vi "translatePolarityValues.vi"(0 "SingleAxisController in":refnum<class "_SingleAxisController.lvclass">, 1 "simple_actions":T3, 2 "polarity_value (in)":u32, 3 "polarity_items (in)":T1[](array[typedef]), 5 "error in (no error)":errorcluster) -> (14 "SingleAxisController out":refnum<class "_SingleAxisController.lvclass">, 16 "polarity_value (out)":u32, 17 "polarity_items (out)":T1[](array[typedef]), 19 "error out":errorcluster)   [LabVIEW 2020, in "classes.lvlib" / "_SingleAxisController.lvclass"]
doc: "Produced By:\n\n<B>Kod Integrations, LLC</B>\n4835 Marianne Drive\nMount Airy, MD 21771\nhttp://www.kodintegrations.com\nemail: info@kodintegrations.com\nphone: (240) 687-1288"
uses:
  _SingleAxisController.lvclass
  common/controls/simple_actions.ctl
  common/controls/polarity_item.ctl
  common/controls/polarity.ctl
  libraries/common.lvlib
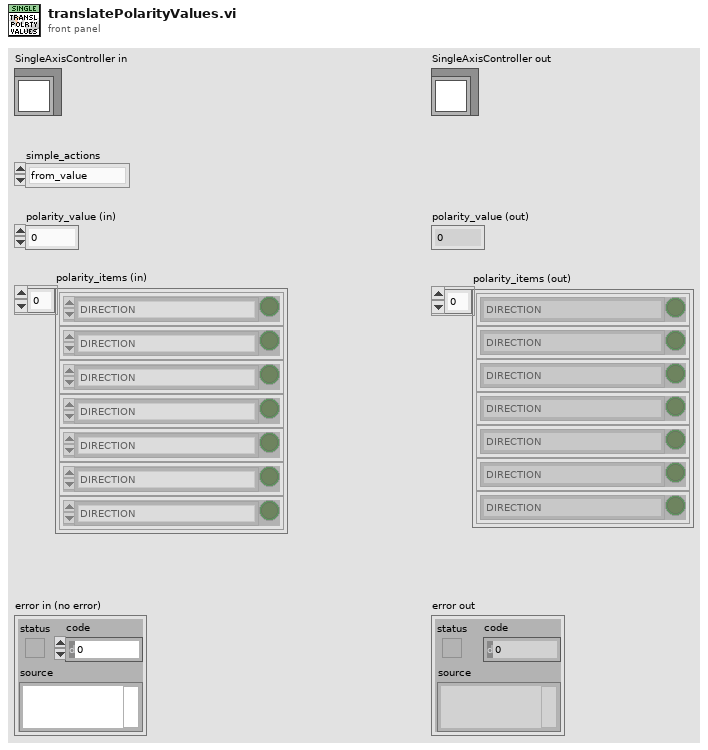
[diagram p1: front panel]
types:
  T1 = typedef "common.lvlib/polarity_item.ctl" = cluster{"item":T2, "status":bool}
  T2 = typedef "common.lvlib/polarity.ctl" = enum16{"DIRECTION", "LIMIT", "HOME", "DIG_OUT", "DIG_IN", "ENABLE_OUT", "JUMP_ERR", "LATCH", "Z-CHAN_INDEX", "ENCODER_DECODING:1X", "ENCODER_DECODING:2X", "ENCODER_DECODING:4X", "ALARM", "STANDALONE_ERR", "-", "<reserved/nc>"}
  T3 = typedef "common.lvlib/simple_actions.ctl" = enum16{"from_value", "to_value"}
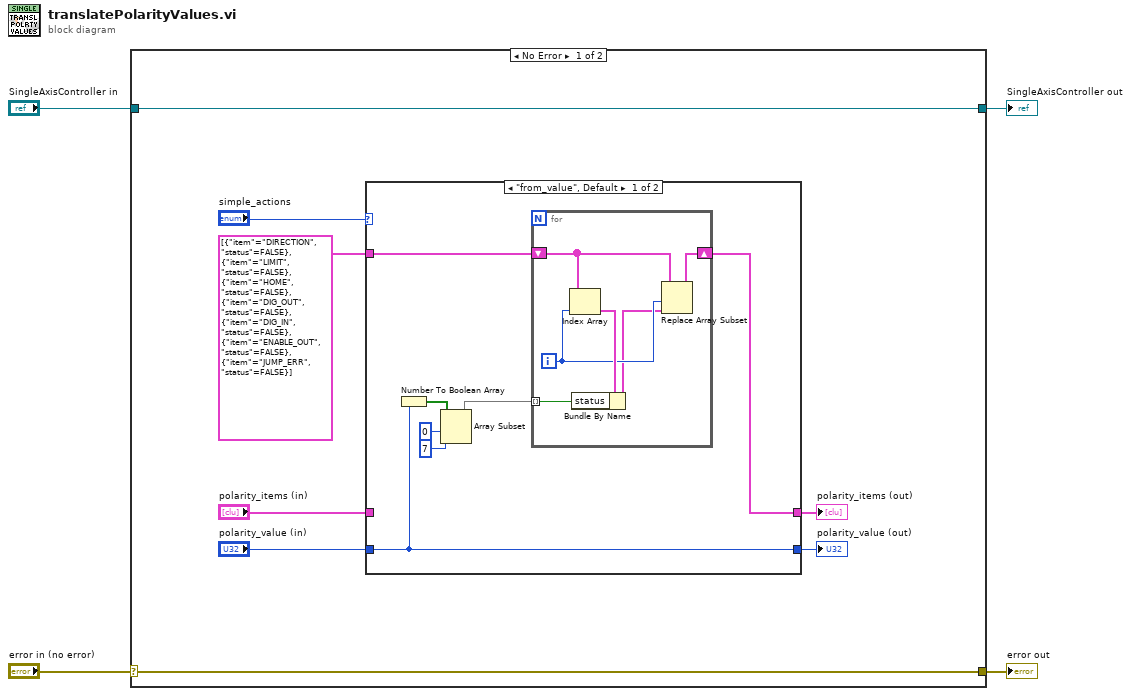
[diagram p0: block diagram]
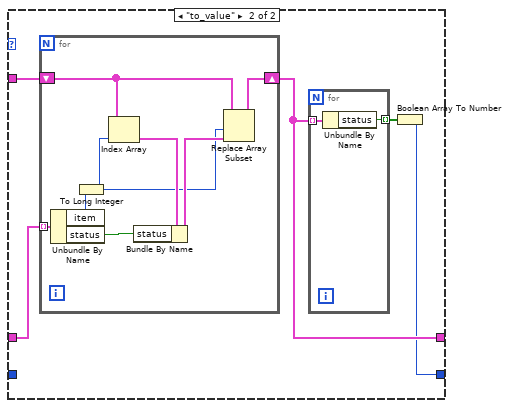
[diagram p2: hidden frame]
diagram:
  n1 = case shown="No Error" "error in (no error)" {
    selector: "error in (no error)" -> [w11 w42]
    tunnel: [w11 w42] -> w3
    tunnel: [w12 w41] -> w1
    tunnel: "SingleAxisController in" -> [w12 w41]
    frame No Error {
      n2 = case shown="\"from_value\", Default" "simple_actions" {
        tunnel: "polarity_value (in)" -> [w13 _]
        tunnel: [w15 w28] -> w8
        tunnel: T1[] [{"item"=enum."DIRECTION", "status"=FALSE}, {"item"=enum."LIMIT", "status"=FALSE}, {"item"=enum."HOME", "status"=FALSE}, {"item"=enum."DIG_OUT", "status"=FALSE}, {"item"=enum."DIG_IN", "status"=FALSE}, {"item"=enum."ENABLE_OUT", "status"=FALSE}, {"item"=enum."JUMP_ERR", "status"=FALSE}] ("polarity_items (in)") -> [w14 w30]
        tunnel: "polarity_items (in)" -> [_ w29]
        tunnel: [w13 w26] -> w5
        frame "from_value", Default {
          n3 = Number To Boolean Array(number=w13) -> (Boolean array=w19:bool[])
          n4 = Array Subset(array=w19, index=0, length=7) -> (w16:bool[])
          n5 = for {
            shift-right: [w20] -> w15
            shift-left: w14 -> [w23]
            tunnel: w16 -> [w24] mode=indexing
            i -> [w22]
            n6 = Index Array(array=w23, index=w22) -> (element=w25:T1)
            n7 = Bundle By Name(cluster=w25, "status"=w24) -> (w21:T1)
            n8 = Replace Array Subset(array=w23, new element=w21, index=w22) -> (w20:T1[])
          }
        }
        frame "to_value" {
          n9 = for {
            shift-right: [w34] -> w28
            shift-left: w30 -> [w33]
            tunnel: w29 -> [w38] mode=indexing
            n10 = Unbundle By Name(w38) -> ("item"=w37:T2, "status"=w36:bool)
            n11 = To Long Integer(number=w37) -> (32bit integer=w35:i32)
            n12 = Index Array(array=w33, index=w35) -> (element=w39:T1)
            n13 = Bundle By Name(cluster=w39, "status"=w36) -> (w40:T1)
            n14 = Replace Array Subset(array=w33, new element=w40, index=w35) -> (w34:T1[])
          }
          n15 = for {
            tunnel: w28 -> [w32] mode=indexing
            tunnel: [w31] -> w27 mode=indexing
            n16 = Unbundle By Name(w32) -> ("status"=w31:bool)
          }
          n17 = Boolean Array To Number(Boolean array=w27) -> (number=w26:u32)
        }
      }
      "polarity_items (out)" <- w8
      "polarity_value (out)" <- w5
    }
    frame Error {
    }
  }
  "error out" <- w3
  "SingleAxisController out" <- w1
